vi "Power Spectrum (DBL).vi"(0 "X":dbl[](array[numeric])) -> (1 "Power Spectrum":dbl[](array[numeric]), 2 "error":i32)   [LabVIEW 2018, in "NI_AALPro.lvlib"]
doc: "Computes the <B>Power Spectrum</B>, Sxx, of the input sequence <B>X</B>. Wire data to the <B>X</B> input to determine the polymorphic instance to use or manually select the instance."
uses:
  <vilib>/Analysis/NI_AALPro.lvlib
  <resource>/lvanlys.dll
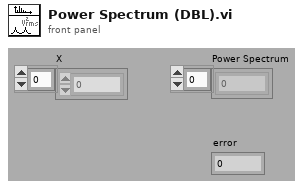
[diagram p1: front panel]
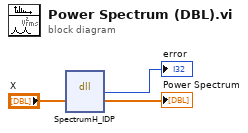
[diagram p0: block diagram]
diagram:
  n1 = dll-call lib="C:/Program Files (x86)/National Instruments/LabVIEW 2018/resource/lvanlys.*" fn="SpectrumH_IDP"("xH"="X") -> ("return type"=→"error":i32, "xH"=→"Power Spectrum":dbl[])  [unwired: 5 in, 2 out]
